vi "example.vi"() -> ()   [LabVIEW 2017]
uses:
  asdk.lib/ASDK.lvlib
panel:
  in  "Serial Name":string
  out "Number of actuators":u32
  out "Initial sent values":dbl[](array[numeric])
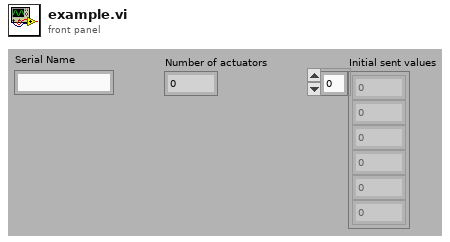
[diagram p1: front panel]
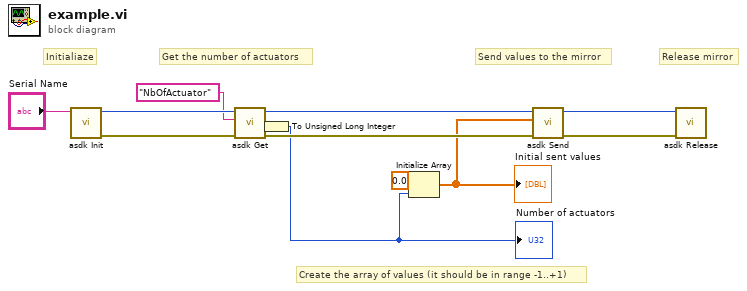
[diagram p0: block diagram]
diagram:
  # "Release mirror"
  # "Send values to the mirror"
  # "Create the array of values (it should be in range -1..+1)"
  # "Get the number of actuators"
  # "Initialiaze"
  n1 = call "asdk Init.vi"("serialName"="Serial Name") -> ("error out"=w11:errorcluster, "function return"=w12:u64)  [unwired: 9 in]
  n2 = call "asdk Get.vi"("error in (no error)"=w11, "command"="NbOfActuator", "pDm"=w12) -> ("error out"=w5:errorcluster, "value out"=w9:dbl, "pDm out"=w6:u64)  [unwired: 6 in]
  n3 = To Unsigned Long Integer(number=w9) -> (unsigned 32bit integer=w3:u32)
  "Number of actuators" <- w3
  n4 = Initialize Array(0.0 ("element"), w3) -> (w4:dbl[])
  "Initial sent values" <- w4
  n5 = call "asdk Send.vi"("error in (no error)"=w5, "value"=w4, "pDm"=w6) -> ("error out"=w8:errorcluster, "pDm out"=w7:u64)  [unwired: 7 in]
  n6 = call "asdk Release.vi"("error in (no error)"=w8, "pDm"=w7) -> ()  [unwired: 9 in, 1 out]
